vi "LVClass_WavefrontCorrectorSet Get Default WavefrontCorrectorParametersSetup.vi"(0 "CameraSet in":refnum<class "WavefrontCorrectorSet.lvclass">, 11 "error in (no error)":errorcluster) -> (4 "CameraSet out":refnum<class "WavefrontCorrectorSet.lvclass">, 15 "error out":errorcluster)   [LabVIEW 2020, in "WavefrontCorrectorSet.lvclass"]
uses:
  WavefrontCorrectorSet.lvclass
  CameraParametersSetup.ctl
  CameraParameters_Type.ctl
  WavefrontCorrectorSet.lvclass/WavefrontCorrectorSet.ctl
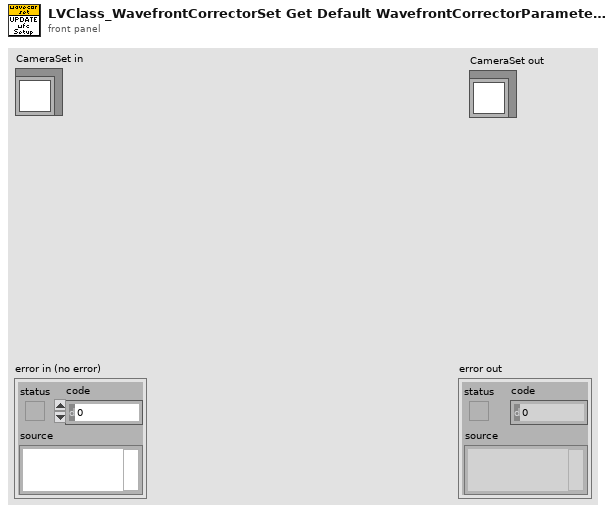
[diagram p1: front panel]
types:
  T1 = typedef "CameraParametersSetup.ctl" = cluster{"Name":string, "Type":T2, "Value":dbl, "BooleanValue":bool, "StringValue":string}
  T2 = typedef "CameraParameters_Type.ctl" = enum16{"Integer", "Real", "String", "Boolean"}
  T3 = typedef "ParameterID.ctl" = cluster{"Name":string, "Type":T2, "Authorization":T4, "OnFlyAuthorization":T5, "StringDefault":string, "Default":dbl, "Min":dbl, "Max":dbl, "Boolean":bool, "StringParameterList":string[]}
  T4 = typedef "CameraParameters_Authorization.ctl" = enum16{"Disable", "Gettable", "Settable - Gettable"}
  T5 = typedef "CameraParameters_OnFlyAuthorization.ctl" = enum16{"None", "Gettable", "Settable", "Settable - Gettable"}
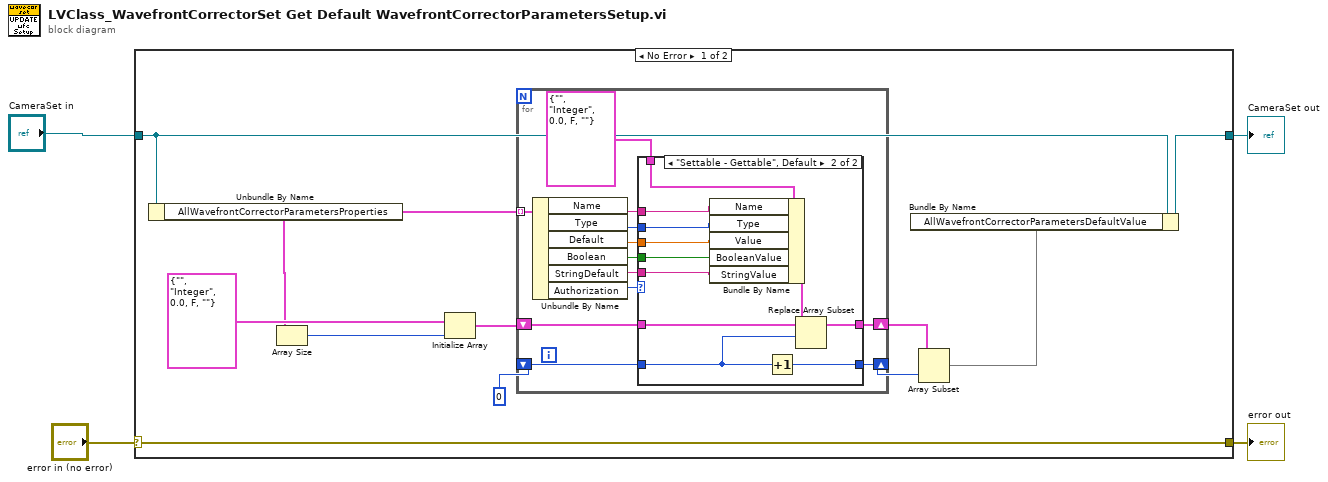
[diagram p0: block diagram]
diagram:
  n1 = case shown="No Error" "error in (no error)" {
    selector: "error in (no error)" -> [w15 w42]
    tunnel: [w15 w42] -> w3
    tunnel: [w7 w41] -> w1
    tunnel: "CameraSet in" -> [w5 w41]
    frame No Error {
      n2 = Unbundle By Name(w5) -> ("AllWavefrontCorrectorParametersProperties"=w9:T3[])
      n3 = Array Size(array=w9) -> (size(s)=w14:i32)
      n4 = Initialize Array(T1 {"Name"="", "Type"=enum."Integer", "Value"=0.0, "BooleanValue"=FALSE, "StringValue"=""} ("CameraParametersSetup"), w14) -> (w10:T1[])
      n5 = for {
        tunnel: w9 -> [w25] mode=indexing
        shift-right: [w26] -> w6
        shift-left: w10 -> [w27]
        shift-right: [w18] -> w12
        shift-left: 0 -> [w17]
        n6 = Unbundle By Name(w25) -> ("Name"=w23:string, "Type"=w22:T2, "Default"=w21:dbl, "Boolean"=w20:bool, "StringDefault"=w19:string, "Authorization"=w16:T4)
        n7 = case shown="\"Settable - Gettable\", Default" w16 {
          tunnel: w27 -> [w29 w40]
          tunnel: [w29 w39] -> w26
          tunnel: T1 {"Name"="", "Type"=enum."Integer", "Value"=0.0, "BooleanValue"=FALSE, "StringValue"=""} ("CameraParametersSetup") -> [_ w37]
          tunnel: w23 -> [_ w36]
          tunnel: w22 -> [_ w35]
          tunnel: w21 -> [_ w34]
          tunnel: w20 -> [_ w33]
          tunnel: w19 -> [_ w32]
          tunnel: [w28 w31] -> w18
          tunnel: w17 -> [w28 w30]
          frame "Disable" {
          }
          frame "Settable - Gettable", Default {
            n8 = Bundle By Name(cluster=w37, "Name"=w36, "Type"=w35, "Value"=w34, "BooleanValue"=w33, "StringValue"=w32) -> (w38:T1)
            n9 = Increment(x=w30) -> (x+1=w31:i32)
            n10 = Replace Array Subset(array=w40, new element=w38, index=w30) -> (w39:T1[])
          }
        }
      }
      n11 = Array Subset(array=w6, length=w12) -> (w8:T1[])  [unwired: 1 in]
      n12 = Bundle By Name(cluster=w5, "AllWavefrontCorrectorParametersDefaultValue"=w8) -> (w7:refnum<class "WavefrontCorrectorSet.lvclass">)
    }
    frame Error {
    }
  }
  "error out" <- w3
  "CameraSet out" <- w1
